vi "Exemple_Model_Selection_LeavePGroupsOut.vi"() -> ()   [LabVIEW 2020]
panel:
  out "Split":T1(array[cluster])
  out "error out":errorcluster caption="sortie d'erreur"
  in  "LeavePGroupsOut":cluster{"n_groups":i32}={"n_groups"=2}
  in  "error in (no error)":errorcluster caption="entrée d'erreur (pas d'erreur)"
  in  "Groups":string[][](array[string])=[["1"], ["2"], ["3"]]
  in  "y":string[][](array[string])=[["1"], ["2"], ["1"]]
  in  "X":string[][](array[string])=[["1", "2"], ["3", "4"], ["5", "6"]]
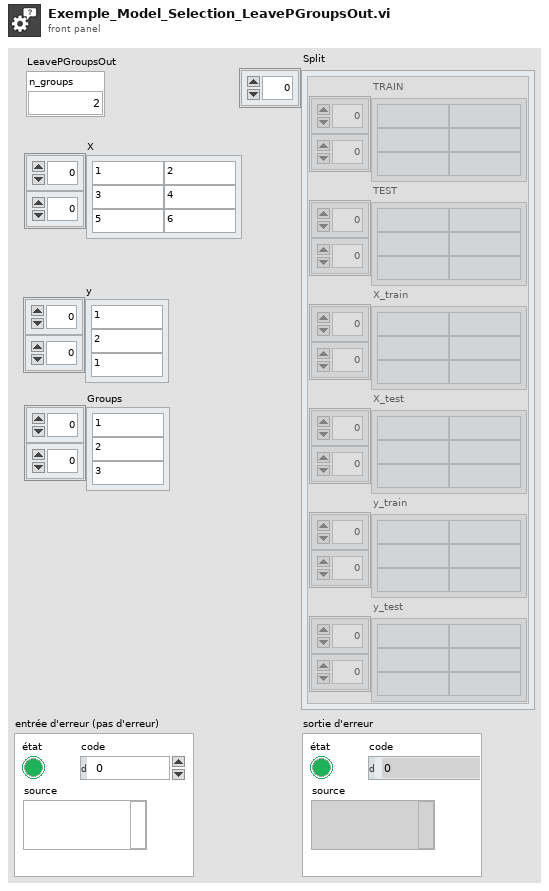
[diagram p1: front panel]
types:
  T1 = cluster{"TRAIN":string[][], "TEST":string[][], "X_train":string[][], "X_test":string[][], "y_train":string[][], "y_test":string[][]}[]
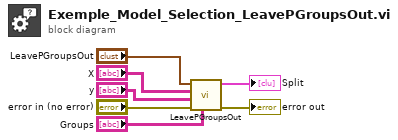
[diagram p0: block diagram]
diagram:
  n1 = call "LeavePGroupsOut.vi"("Groups"="Groups", "error in (no error)"="error in (no error)", "y"="y", "X"="X", "LeavePGroupsOut"="LeavePGroupsOut") -> ("error out"=→"error out":errorcluster, "Split"=→"Split":T1)  [unwired: 5 in]
